vi "TransducerTypeInformation.vi"(8 "error in (no error)":errorcluster, 11 "Connection Data In":T2) -> (0 "error out":errorcluster, 2 "Cluster Calibration":T1, 3 "Connection Data Out":T2)   [LabVIEW 2014, in "MSX-E3701_dll.lvlib"]
doc: "Recorre la memoria del Data base buscando la información de los transductores que esta misma aloja, adquiere la información de cada uno y los envía al Clúster de Calibración."
uses:
  MSX-E3701_dll.lvlib
  Typedef/Connection Data.ctl
  E:/Repositorio Magnis/INF002/v0/Modules/HAL/Drivers/Sync/ADDI-DATA MSX-E3701/API/MX370x.dll
  MX370x.dll
  E:/Repositorio Magnis/INF002/v0/Modules/HAL/Drivers/Sync/ADDI-DATA MSX-E3701/API/MXCommon.dll
  MXCommon.dll
  Typedef/Calibration Data.ctl
panel:
  # "Information"
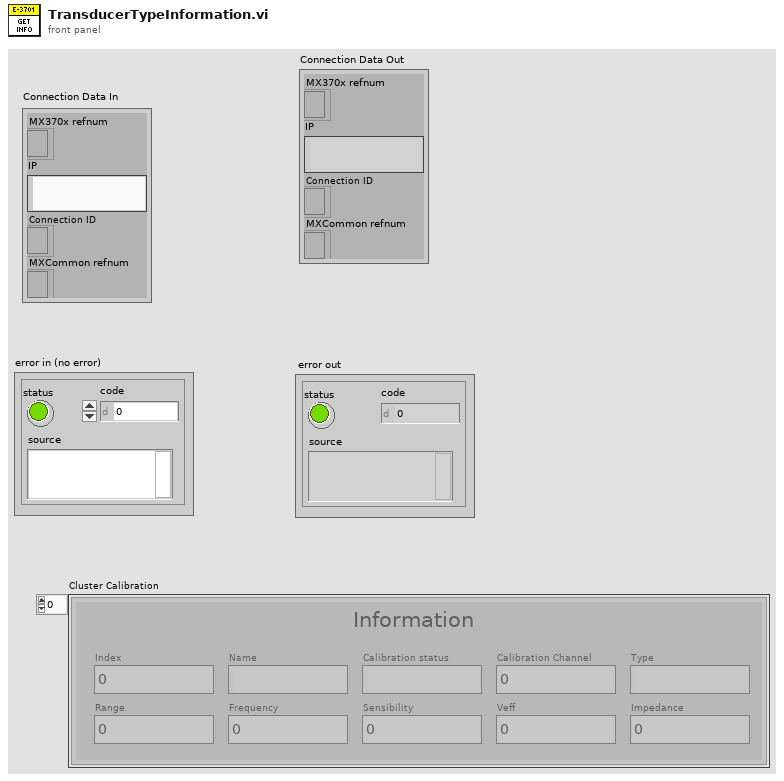
[diagram p1: front panel]
types:
  T1 = typedef "MSX-E3701_dll.lvlib/Calibration Data.ctl" = cluster{"Calibration status":string, "Name":string, "Index":u64, "Range":dbl, "Sensibility":dbl, "Veff":dbl, "Frequency":u64, "Impedance":u64, "Type":string, "Calibration Channel":u64}[]
  T2 = typedef "MSX-E3701_dll.lvlib/Connection Data.ctl" = cluster{"MX370x refnum":refnum<k24>, "IP":string, "Connection ID ":refnum<k5>, "MXCommon refnum":refnum<k24>}
  T3 = cluster{"Calibration status":string, "Name":string, "Index":u64, "Range":dbl, "Sensibility":dbl, "Veff":dbl, "Frequency":u64, "Impedance":u64, "Type":string, "Calibration Channel":u64}
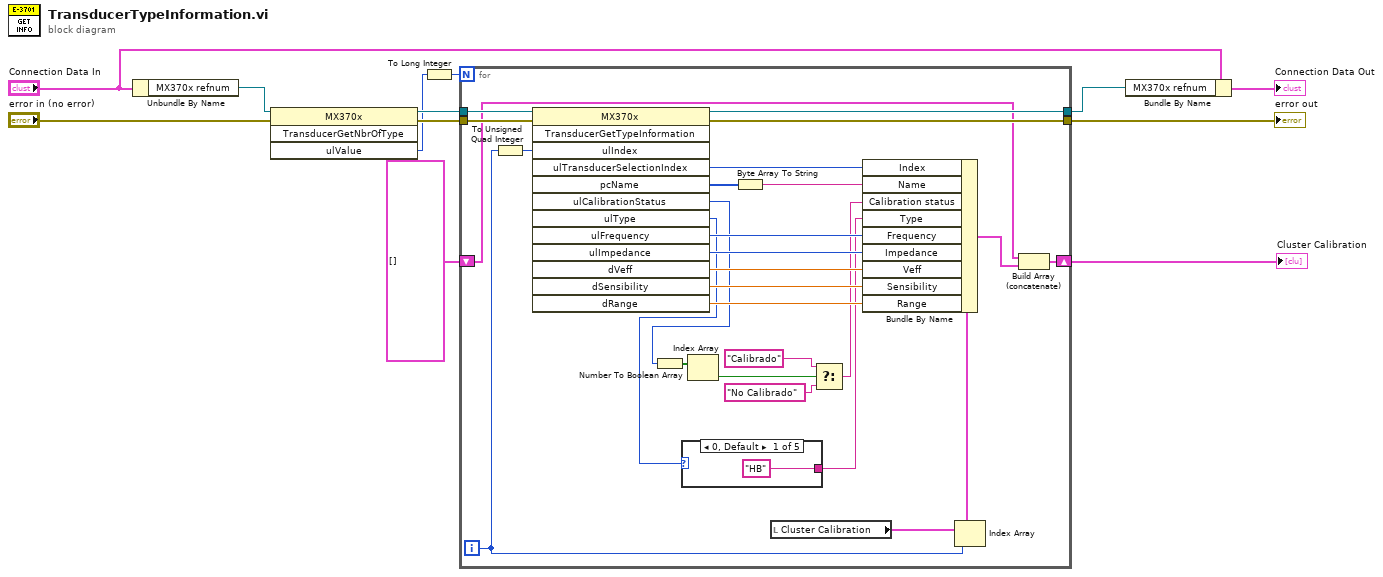
[diagram p0: block diagram]
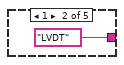
[diagram p2: hidden frame]
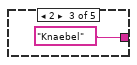
[diagram p3: hidden frame]
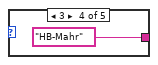
[diagram p4: hidden frame]
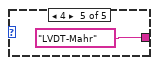
[diagram p5: hidden frame]
diagram:
  n1 = Unbundle By Name("Connection Data In") -> ("MX370x refnum"=w11:refnum<k24>)
  n2 = invoke class="MX370x" method="TransducerGetNbrOfType"(reference=w11, error in="error in (no error)") -> (reference out=w8:refnum<k24>, error out=w7:errorcluster, "ulValue"=w4:u64)  [unwired: 2 in, 1 out]
  n3 = To Long Integer(number=w4) -> (32bit integer=w5:i32)
  n4 = for {
    N: w5 -> [_]
    tunnel: w8 -> [w39]
    tunnel: w7 -> [w38]
    tunnel: [w37] -> w3
    tunnel: [w36] -> w6
    shift-right: [w22] -> w2
    shift-left: T1 [] ("Cluster Calibration 2") -> [w21]
    i -> [w24]
    n5 = To Unsigned Quad Integer(1:w24) -> (0:w35:u64)
    n6 = invoke class="MX370x" method="TransducerGetTypeInformation"(reference=w39, error in=w38, "ulIndex"=w35) -> (reference out=w37:refnum<k24>, error out=w36:errorcluster, "ulTransducerSelectionIndex"=w33:u64, "pcName"=w34:u8[], "ulCalibrationStatus"=w16:u64, "ulType"=w14:u64, "ulFrequency"=w31:u64, "ulImpedance"=w30:u64, "dVeff"=w29:dbl, "dSensibility"=w28:dbl, "dRange"=w27:dbl)  [unwired: 10 in, 2 out]
    n7 = Number To Boolean Array(number=w16) -> (Boolean array=w17:bool[])
    n8 = case shown="0, Default" w14 {
      tunnel: ["HB" "LVDT" "Knaebel" "HB-Mahr" "LVDT-Mahr"] -> w13
      frame 0, Default {
      }
      frame 1 {
      }
      frame 2 {
      }
      frame 3 {
      }
      frame 4 {
      }
    }
    n9 = Index Array(array=w17) -> (element=w15:bool)  [unwired: 1 in]
    n10 = Byte Array To String(unsigned byte array=w34) -> (string=w32:string)
    n11 = local read "Cluster Calibration"() -> (w26:T1)
    n12 = Select(t="Calibrado", s=w15, f="No Calibrado") -> (s? t:f=w20:string)
    n13 = Index Array(array=w26, index=w24) -> (element=w25:T3)
    n14 = Bundle By Name(cluster=w25, "Index"=w33, "Name"=w32, "Calibration status"=w20, "Type"=w13, "Frequency"=w31, "Impedance"=w30, "Veff"=w29, "Sensibility"=w28, "Range"=w27) -> (w23:T3)
    n15 = Build Array (concatenate)(w21, w23) -> (w22:T1)
  }
  "error out" <- w6
  "Cluster Calibration" <- w2
  n16 = Bundle By Name(cluster="Connection Data In", "MX370x refnum"=w3) -> (→"Connection Data Out":T2)
